vi "JSON Array to Display Text.vi"(10 "Array of JSON Text":string[](array[string])) -> (3 "Display Text":string)   [LabVIEW 2017, in "JSONtext.lvlib"]
uses:
  JSONtext.lvlib
  <vilib>/JDP Science/JDP Science Common Utilities/Trim Whitespace__JDP.vi
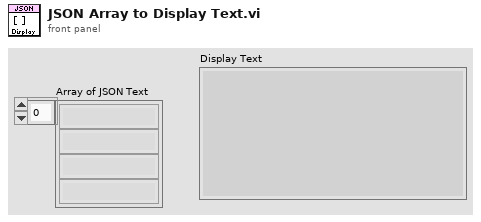
[diagram p1: front panel]
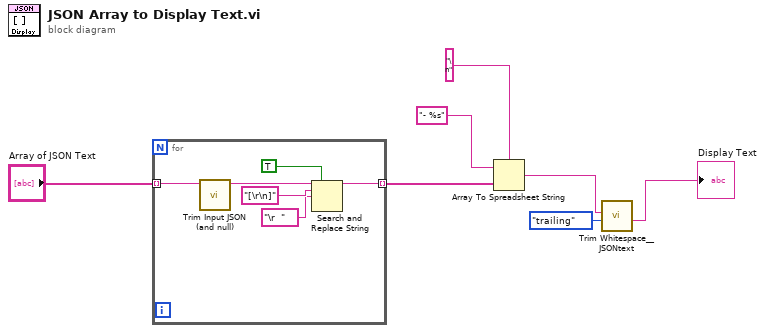
[diagram p0: block diagram]
diagram:
  n1 = for {
    tunnel: "Array of JSON Text" -> [w13] mode=indexing
    tunnel: [w8] -> w4 mode=indexing
    n2 = call "Trim Input JSON (and null).vi"("JSON Input"=w13) -> ("<JSON>"=w11:string)  [unwired: 10 in]
    n3 = Search and Replace String(replace all?=TRUE ("replace all? (F)"), input string=w11, search string="[\r\n]", replace string="\r  " ("search string")) -> (result string=w8:string)  [unwired: 4 in, 3 out]
  }
  n4 = Array To Spreadsheet String(delimiter (Tab)="\n", array=w4, 3:"- %s" ("format string")) -> (spreadsheet string=w2:string)
  n5 = call "Trim Whitespace__JSONtext.vi"("Remove (leading and trailing)"=enum16{"leading", "trailing", "both"}."trailing", "String in"=w2) -> ("String out"=→"Display Text":string)  [unwired: 5 in]
